vi "PH_Countdown-Counter.PC LastShot.vi"(0 "i ref in":refnum<vi>, 2 "Servicename":string, 3 "Last Shot":timestamp, 4 "no link?":bool, 5 "error in (no error)":errorcluster) -> (14 "i ref out":refnum<vi>, 19 "error out":errorcluster)   [LabVIEW 2014, in "PH_Countdown-Counter.lvlib"]
doc: "This VI writes the remaining waiting time of the PU to own attributes and the GUI elements."
uses:
  PH_Countdown-Counter.lvlib
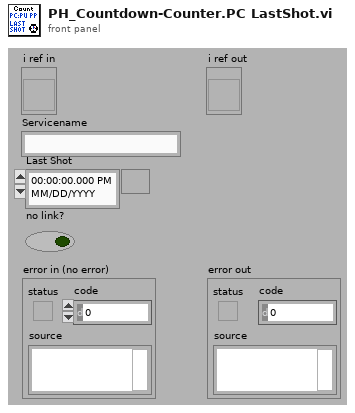
[diagram p1: front panel]
types:
  T1 = typedef "PH_Countdown-Counter.lvlib/PH_Countdown-Counter.i attribute.ctl" = cluster{"Machine Time":cluster{"Tag":string, "Wating Time [s]":dbl, "not linked?":bool}[], "Last Shot":cluster{"Tag":string, "Shot Time [s]":timestamp, "not linked?":bool}[], "Time since last Shot?":bool, "Calculation":cluster{"Time between Shots [s]":dbl, "Ref Remaining Time":refnum<vi>, "Service ID":i32, "over?":bool, "Ref Time between Shots":refnum<vi>, "Ref Set Mode":refnum<vi>}, "Sound?":bool, "Reminder":cluster{"# 1":cluster{"Pretime [s]":dbl, "Aktive?":bool, "Over?":bool}, "# 2":cluster{"Pretime [s]":dbl, "Aktive?":bool, "Over?":bool}}, "MainAmp only":cluster{"State":bool, "GUI Ref":refnum<vi>}}
  T2 = cluster{"Tag":string, "Shot Time [s]":timestamp, "not linked?":bool}[]
  T3 = cluster{"Tag":string, "Shot Time [s]":timestamp, "not linked?":bool}
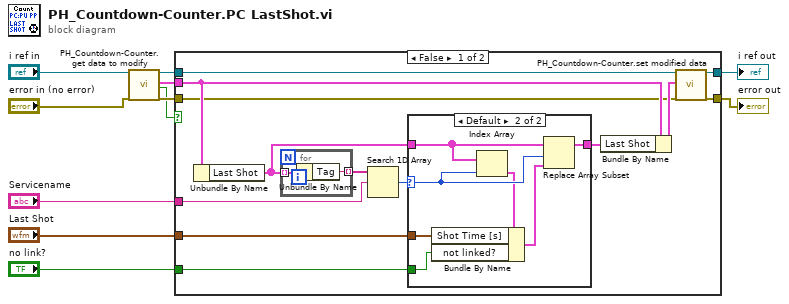
[diagram p0: block diagram]
diagram:
  n1 = call "PH_Countdown-Counter.get data to modify.vi"("i ref in"="i ref in", "error in (no error)"="error in (no error)") -> ("i ref out"=w7:refnum<vi>, "i attribute"=w4:T1, "timed out"=w1:bool, "error out"=w10:errorcluster)  [unwired: 14 in]
  n2 = case shown="False" w1 {
    tunnel: "Last Shot" -> [w13 _]
    tunnel: w10 -> [w12 w35]
    tunnel: w7 -> [w24 w36]
    tunnel: "Servicename" -> [w22 _]
    tunnel: "no link?" -> [w20 _]
    tunnel: w4 -> [w18 _]
    tunnel: [w16 w36] -> w3
    tunnel: [w14 w35] -> w2
    frame False {
      n3 = Unbundle By Name(w18) -> ("Last Shot"=w19:T2)
      n4 = for {
        tunnel: w19 -> [w34] mode=indexing
        tunnel: [w33] -> w23 mode=indexing
        n5 = Unbundle By Name(w34) -> ("Tag"=w33:string)
      }
      n6 = Search 1D Array(1D array=w23, element=w22) -> (index of element=w21:i32)  [unwired: 1 in]
      n7 = case shown="Default" w21 {
        selector: w21 -> [_ w27]
        tunnel: w13 -> [_ w32]
        tunnel: w20 -> [_ w29]
        tunnel: w19 -> [w25 w28]
        tunnel: [w25 w30] -> w17
        frame -1 {
        }
        frame Default {
          n8 = Index Array(array=w28, index=w27) -> (element=w26:T3)
          n9 = Bundle By Name(cluster=w26, "Shot Time [s]"=w32, "not linked?"=w29) -> (w31:T3)
          n10 = Replace Array Subset(array=w28, new element=w31, index=w27) -> (w30:T2)
        }
      }
      n11 = Bundle By Name(cluster=w18, "Last Shot"=w17) -> (w15:T1)
      n12 = call "PH_Countdown-Counter.set modified data.vi"("i ref in"=w24, "i attribute"=w15, "error in (no error)"=w12) -> ("i ref out"=w16:refnum<vi>, "error out"=w14:errorcluster)  [unwired: 15 in]
    }
    frame True {
    }
  }
  "error out" <- w2
  "i ref out" <- w3
